vi "RecognitionSystem).vi"() -> ()   [LabVIEW 2011]
uses:
  <vilib>/DAQmx/read.llb/DAQmx Read (Digital Bool 1Line 1Point).vi
  <vilib>/DAQmx/write.llb/DAQmx Write (Digital Bool 1Line 1Point).vi
  <vilib>/DAQmx/create/channels.llb/DAQmx Create Channel (DI-Digital Input).vi
  <vilib>/DAQmx/create/channels.llb/DAQmx Create Channel (DO-Digital Output).vi
  <vilib>/DAQmx/miscellaneous.llb/DAQmx Fill In Error Info.vi
  <vilib>/Utility/file.llb/Read From Spreadsheet File (string).vi
  <vilib>/Utility/file.llb/Write To Spreadsheet File (string).vi
panel:
  in  "Tab Control":enum32{"System", "Sensors & Actuators"}(tab)
  in  "Data - File Path":path
  in  "Queue - File Path":path
  out "System Efficiency":dbl(knob) scale=0.0..100.0
  in  "Pause":bool
  out "Metal Count":dbl
  out "Plastic Count":dbl
  out "Dequeued Element":string
  out "# Elements in Queue":i32
  out "Hopper \nCount":i32(slide) scale=0.0..5.0
  in  "Stop GUI":bool
  out "Running":bool
  out "Stop":bool
  out "Belt & Chain":bool
  out "Assembled":dbl
  out "Efficiency":dbl
  out "Assembled":u8(slide) scale=0.0..10.0
  out "Plastics":u8(slide) scale=0.0..10.0
  out "Metals":u8(slide) scale=0.0..10.0
  out "Infrared Detector":bool
  out "Metal Detector":bool
  out "Sort Solenoid":bool=TRUE
  out "Assembly IR":bool
  out "Rotary Solenoid":bool=TRUE
  out "Reject IR":bool
  out "Sensing - Metal Detector":bool
  out "Capacitive Sensor":bool
  out "Fibre Optic":bool
  out "Reject Solenoid":bool
  out "Metal State":bool=TRUE
  out "Metal State 2":bool
  out "Capacitive State":bool=TRUE
  out "Sensing - Plastic State":bool
  out "Sort Solenoid Return":bool
  out "File Read":bool=TRUE
  out "Loop Iteration":i32
  out "Reject Solenoid Return":bool
  out "Reject IR - Neg Edge":bool
  out "Fibre Optic - Neg Edge":bool
  out "Pos Edge - Capacitive State":bool
  out "Pos Edge - Metal State 2":bool
  out "Fibre Optic Pos Edge":bool
  out "Capacitive - NEG Edge":bool
  out "Positive Edge - Rotary Solenoid":bool
  out "Reject IR - Pos Edge":bool
  out "IR Positive Edge":bool
  out "IR Negative Edge":bool
  # "Not Important Indicators"
  # "ICT Control System"
  # "Assembly Unit"
  # "Data Values"
  # "Rejecting Section"
  # "Sorting Section"
  # "Assembly Section"
  # "Sensing Section"
  # "Sort Solenoid Return"
  # "System States"
  # "File Read"
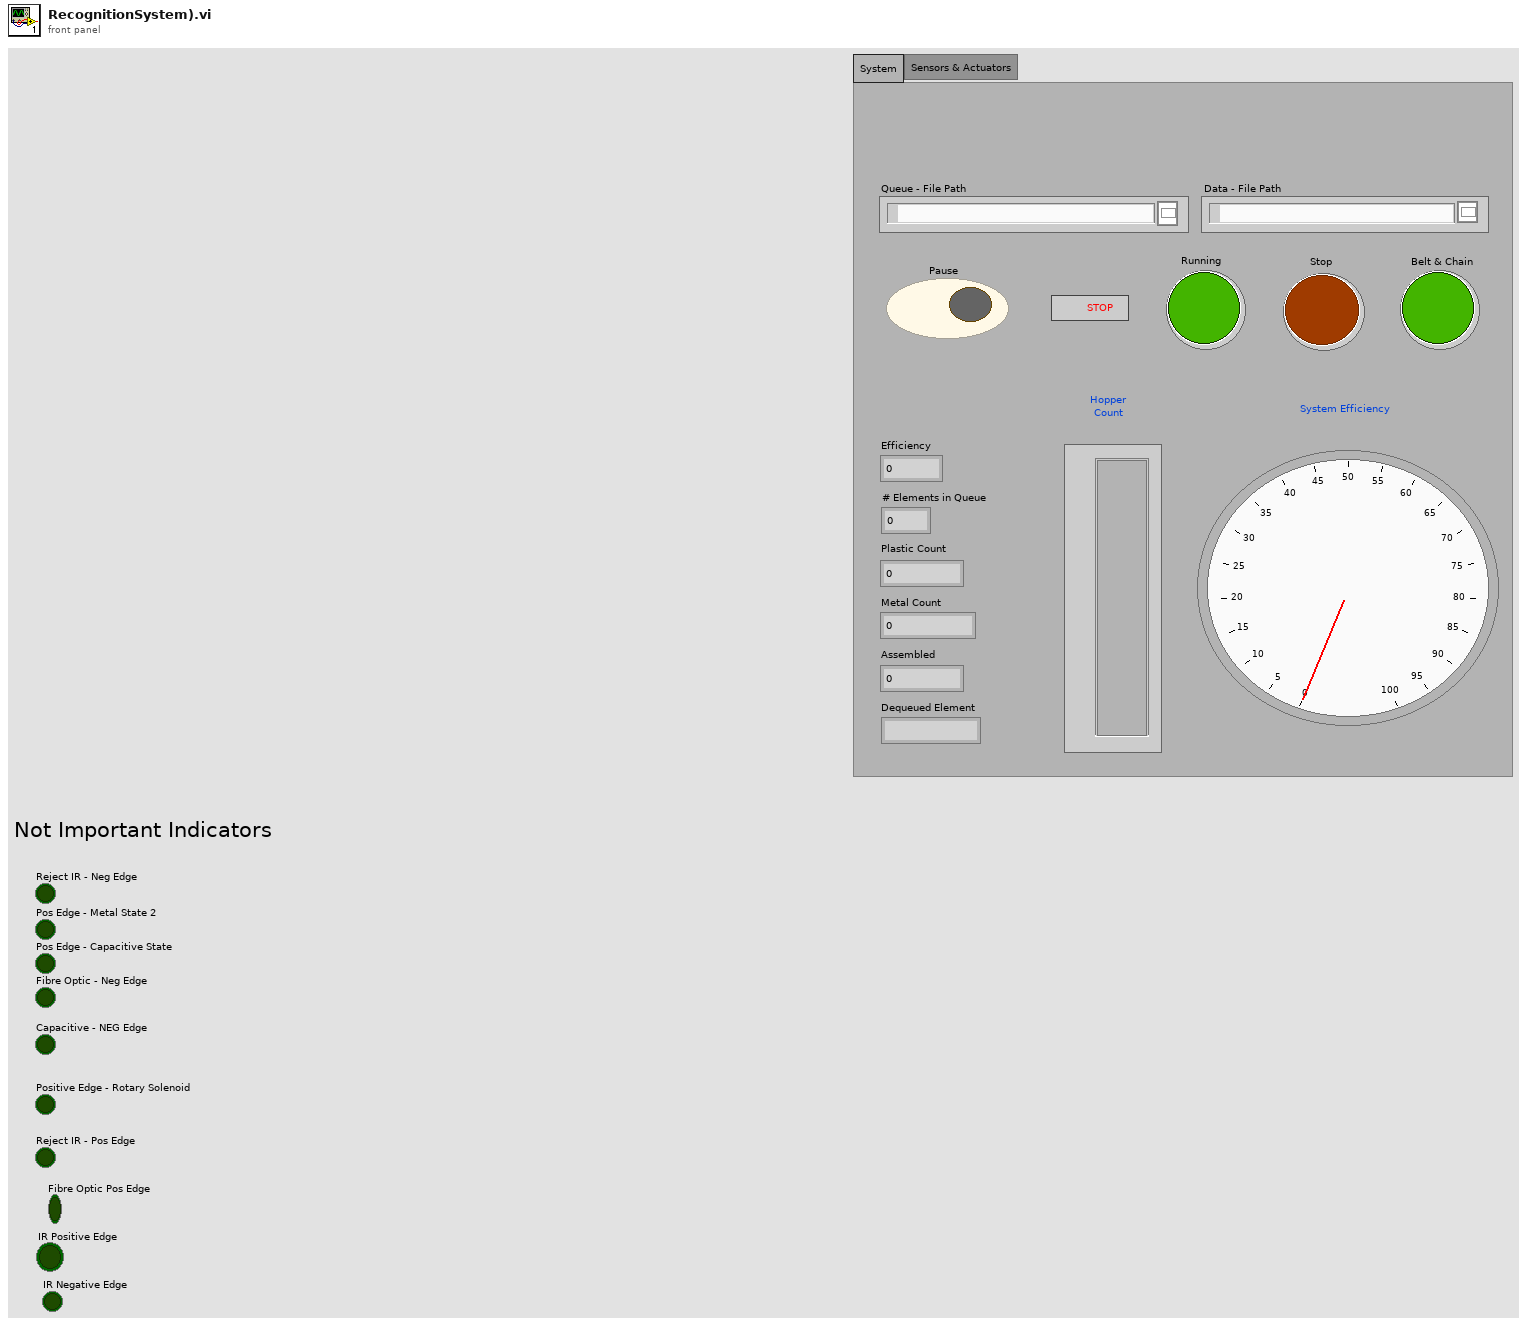
[diagram p1: front panel]
types:
  T1 = enum16{"open", "replace", "create", "open or create", "replace or create", "replace or create with confirmation"}
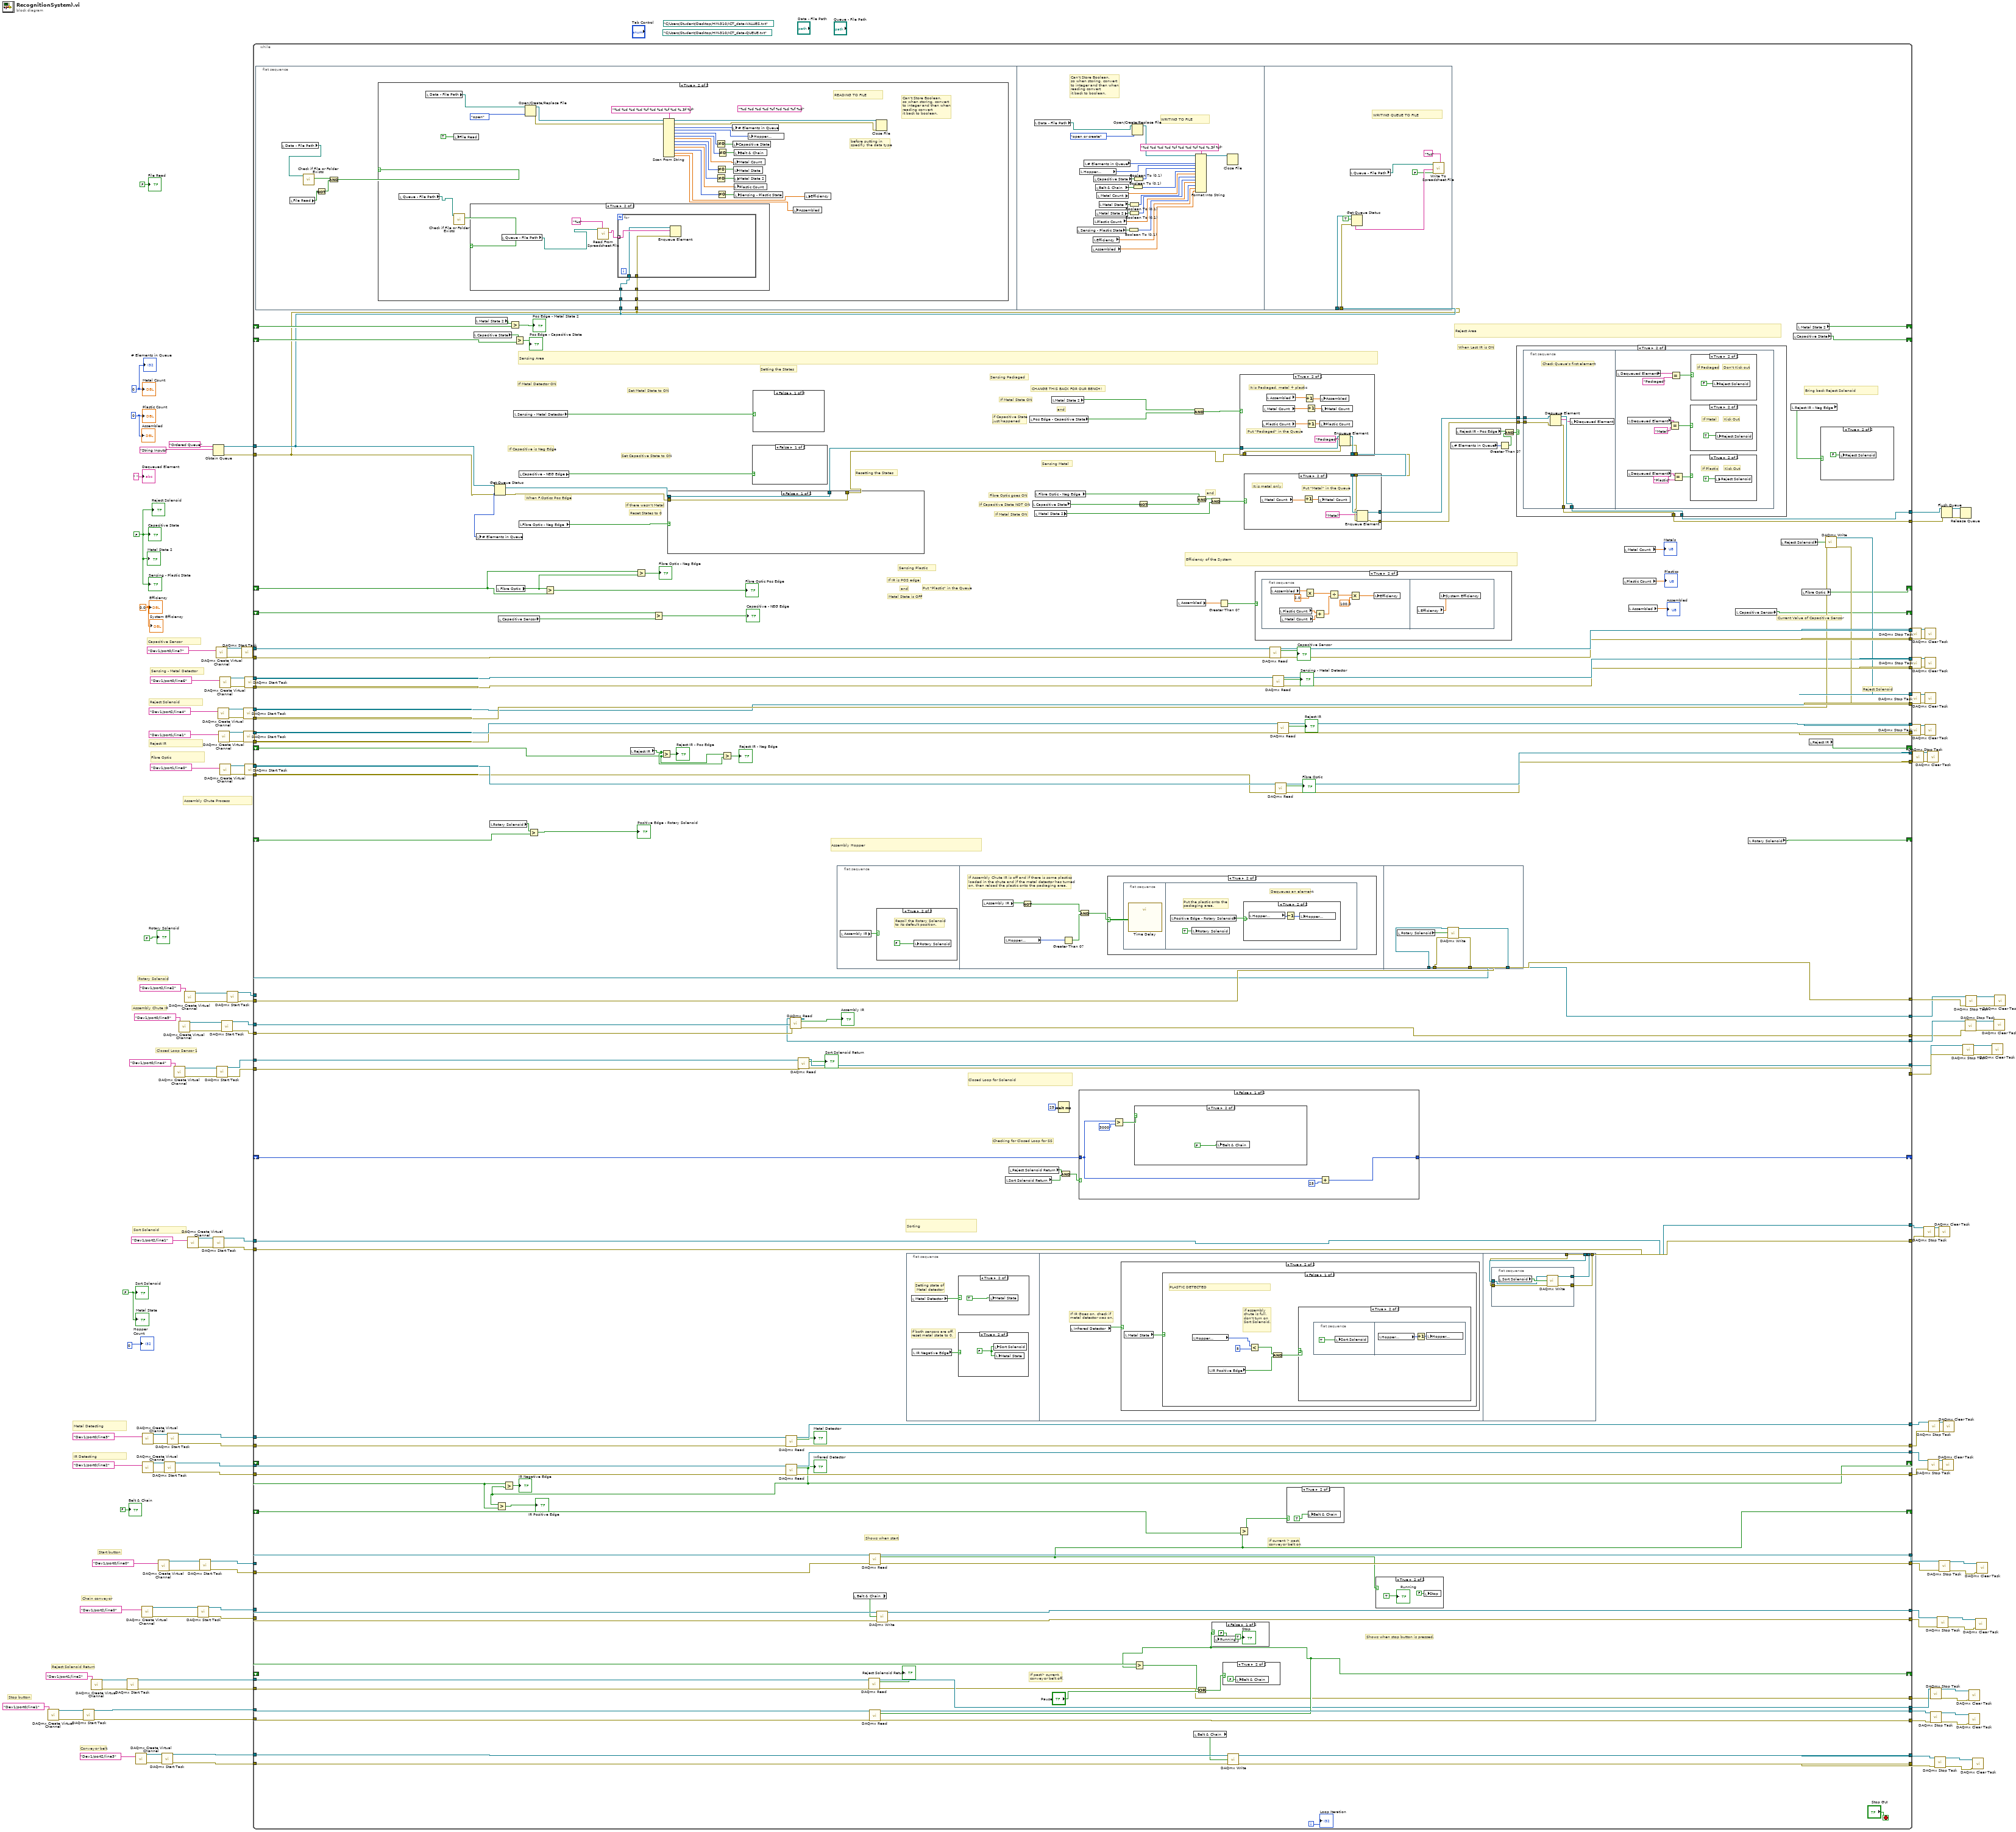
[diagram p0: block diagram]
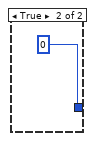
[diagram p3: hidden frame]
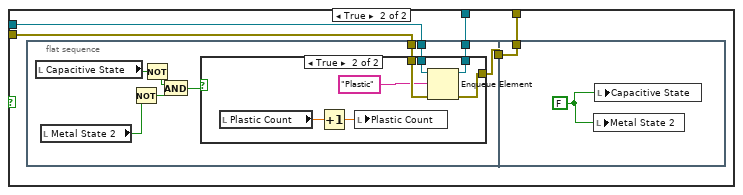
[diagram p16: hidden frame]
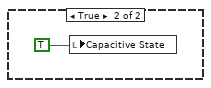
[diagram p18: hidden frame]
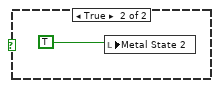
[diagram p19: hidden frame]
diagram:
  (unwired) path "C:/Users/Student/Desktop/HM-310/ICT_data-QUEUE.txt" ("file path (use dialog)")
  (unwired) path "C:/Users/Student/Desktop/HM-310/ICT_data-VALUES.txt" ("file path (use dialog)")
  w10 = 0.0 ("Efficiency")
  w12 = 0
  w15 = 0
  w26 = FALSE
  w25 = FALSE
  # "Reject Solenoid Return"
  # "Conveyor belt"
  # "Fibre Optic"
  # "Assembly Chute Process"
  # "Reject IR"
  # "Reject Solenoid"
  # "Sensing - Metal Detector"
  # "Capacitive Sensor"
  # "Rotary Solenoid"
  # "Assembly Chute IR"
  # "Closed Loop Sensor 1"
  # "Sort Solenoid"
  # "Chain conveyor"
  # "Stop button"
  # "Start button"
  # "IR Detecting"
  # "Metal Detecting"
  n1 = call-poly <vilib>:"DAQmx Create Virtual Channel.vi"("lines"=tag "Dev1/port0/line1") -> ("task out"=w111:refnum<k21>, "error out"=w119:errorcluster)  [unwired: 13 in]
  n2 = call <vilib>:"DAQmx Start Task.vi"("task/channels in"=w111, "error in"=w119) -> ("task out"=w117:refnum<k21>, "error out"=w116:errorcluster)  [unwired: 12 in]
  n3 = call-poly <vilib>:"DAQmx Create Virtual Channel.vi"("lines"=tag "Dev1/port1/line2") -> ("task out"=w7:refnum<k21>, "error out"=w9:errorcluster)  [unwired: 13 in]
  n4 = call <vilib>:"DAQmx Start Task.vi"("task/channels in"=w7, "error in"=w9) -> ("task out"=w2:refnum<k21>, "error out"=w1:errorcluster)  [unwired: 12 in]
  n5 = call-poly <vilib>:"DAQmx Create Virtual Channel.vi"("lines"=tag "Dev1/port2/line3") -> ("task out"=w36:refnum<k21>, "error out"=w35:errorcluster)  [unwired: 13 in]
  n6 = call-poly <vilib>:"DAQmx Create Virtual Channel.vi"("lines"=tag "Dev1/port2/line0") -> ("task out"=w128:refnum<k21>, "error out"=w127:errorcluster)  [unwired: 13 in]
  n7 = call-poly <vilib>:"DAQmx Create Virtual Channel.vi"("lines"=tag "Dev1/port0/line3") -> ("task out"=w161:refnum<k21>, "error out"=w160:errorcluster)  [unwired: 13 in]
  n8 = call-poly <vilib>:"DAQmx Create Virtual Channel.vi"("lines"=tag "Dev1/port0/line2") -> ("task out"=w147:refnum<k21>, "error out"=w146:errorcluster)  [unwired: 13 in]
  n9 = call-poly <vilib>:"DAQmx Create Virtual Channel.vi"("lines"=tag "Dev1/port0/line0") -> ("task out"=w136:refnum<k21>, "error out"=w135:errorcluster)  [unwired: 13 in]
  n10 = call <vilib>:"DAQmx Start Task.vi"("task/channels in"=w36, "error in"=w35) -> ("task out"=w33:refnum<k21>, "error out"=w32:errorcluster)  [unwired: 12 in]
  n11 = call <vilib>:"DAQmx Start Task.vi"("task/channels in"=w147, "error in"=w146) -> ("task out"=w141:refnum<k21>, "error out"=w140:errorcluster)  [unwired: 12 in]
  n12 = call <vilib>:"DAQmx Start Task.vi"("task/channels in"=w161, "error in"=w160) -> ("task out"=w150:refnum<k21>, "error out"=w149:errorcluster)  [unwired: 12 in]
  n13 = call-poly <vilib>:"DAQmx Create Virtual Channel.vi"("lines"=tag "Dev1/port0/line4") -> ("task out"=w108:refnum<k21>, "error out"=w107:errorcluster)  [unwired: 13 in]
  n14 = call-poly <vilib>:"DAQmx Create Virtual Channel.vi"("lines"=tag "Dev1/port0/line5") -> ("task out"=w99:refnum<k21>, "error out"=w98:errorcluster)  [unwired: 13 in]
  n15 = call-poly <vilib>:"DAQmx Create Virtual Channel.vi"("lines"=tag "Dev1/port2/line2") -> ("task out"=w88:refnum<k21>, "error out"=w87:errorcluster)  [unwired: 13 in]
  n16 = call-poly <vilib>:"DAQmx Create Virtual Channel.vi"("lines"=tag "Dev1/port2/line1") -> ("task out"=w157:refnum<k21>, "error out"=w156:errorcluster)  [unwired: 13 in]
  n17 = call <vilib>:"DAQmx Start Task.vi"("task/channels in"=w128, "error in"=w127) -> ("task out"=w125:refnum<k21>, "error out"=w124:errorcluster)  [unwired: 12 in]
  n18 = call <vilib>:"DAQmx Start Task.vi"("task/channels in"=w136, "error in"=w135) -> ("task out"=w134:refnum<k21>, "error out"=w133:errorcluster)  [unwired: 12 in]
  n19 = Obtain Queue(name (unnamed)="Ordered Queue", element data type="String Inputs") -> (queue out=w22:refnum<queue>, error out=w21:errorcluster)  [unwired: 3 in, 1 out]
  n20 = call <vilib>:"DAQmx Start Task.vi"("task/channels in"=w157, "error in"=w156) -> ("task out"=w139:refnum<k21>, "error out"=w138:errorcluster)  [unwired: 12 in]
  n21 = call-poly <vilib>:"DAQmx Create Virtual Channel.vi"("lines"=tag "Dev1/port0/line7") -> ("task out"=w80:refnum<k21>, "error out"=w79:errorcluster)  [unwired: 13 in]
  n22 = call <vilib>:"DAQmx Start Task.vi"("task/channels in"=w108, "error in"=w107) -> ("task out"=w105:refnum<k21>, "error out"=w104:errorcluster)  [unwired: 12 in]
  n23 = call-poly <vilib>:"DAQmx Create Virtual Channel.vi"("lines"=tag "Dev1/port2/line4") -> ("task out"=w74:refnum<k21>, "error out"=w73:errorcluster)  [unwired: 13 in]
  n24 = call-poly <vilib>:"DAQmx Create Virtual Channel.vi"("lines"=tag "Dev1/port1/line1") -> ("task out"=w71:refnum<k21>, "error out"=w70:errorcluster)  [unwired: 13 in]
  n25 = call-poly <vilib>:"DAQmx Create Virtual Channel.vi"("lines"=tag "Dev1/port0/line6") -> ("task out"=w77:refnum<k21>, "error out"=w76:errorcluster)  [unwired: 13 in]
  n26 = call-poly <vilib>:"DAQmx Create Virtual Channel.vi"("lines"=tag "Dev1/port1/line0") -> ("task out"=w60:refnum<k21>, "error out"=w59:errorcluster)  [unwired: 13 in]
  n27 = call <vilib>:"DAQmx Start Task.vi"("task/channels in"=w99, "error in"=w98) -> ("task out"=w96:refnum<k21>, "error out"=w95:errorcluster)  [unwired: 12 in]
  n28 = call <vilib>:"DAQmx Start Task.vi"("task/channels in"=w88, "error in"=w87) -> ("task out"=w85:refnum<k21>, "error out"=w84:errorcluster)  [unwired: 12 in]
  n29 = call <vilib>:"DAQmx Start Task.vi"("task/channels in"=w80, "error in"=w79) -> ("task out"=w69:refnum<k21>, "error out"=w68:errorcluster)  [unwired: 12 in]
  n30 = call <vilib>:"DAQmx Start Task.vi"("task/channels in"=w74, "error in"=w73) -> ("task out"=w65:refnum<k21>, "error out"=w64:errorcluster)  [unwired: 12 in]
  n31 = call <vilib>:"DAQmx Start Task.vi"("task/channels in"=w71, "error in"=w70) -> ("task out"=w63:refnum<k21>, "error out"=w62:errorcluster)  [unwired: 12 in]
  n32 = call <vilib>:"DAQmx Start Task.vi"("task/channels in"=w77, "error in"=w76) -> ("task out"=w67:refnum<k21>, "error out"=w66:errorcluster)  [unwired: 12 in]
  n33 = call <vilib>:"DAQmx Start Task.vi"("task/channels in"=w60, "error in"=w59) -> ("task out"=w58:refnum<k21>, "error out"=w57:errorcluster)  [unwired: 12 in]
  n34 = while {
    tunnel: [w318] -> w152
    tunnel: [w317] -> w151
    tunnel: w150 -> [w316]
    tunnel: w149 -> [w315]
    tunnel: [w314] -> w143
    tunnel: [w313] -> w142
    tunnel: w141 -> [w312]
    tunnel: w140 -> [w311]
    tunnel: w139 -> [w281]
    tunnel: w138 -> [w280]
    tunnel: w134 -> [w308]
    tunnel: w133 -> [w307]
    tunnel: [w306] -> w130
    tunnel: [w305] -> w129
    tunnel: w125 -> [w304]
    tunnel: w124 -> [w303]
    tunnel: [w302] -> w121
    tunnel: [w301] -> w120
    tunnel: w117 -> [w300]
    tunnel: w116 -> [w299]
    tunnel: [w298] -> w113
    tunnel: [w297] -> w112
    shift-right: [w178] -> _
    shift-left: _ -> [w296]
    shift-right: [w179] -> _
    shift-left: _ -> [w294]
    tunnel: [w283] -> w101
    shift-right: [w285] -> _
    shift-left: _ -> [w286]
    tunnel: w105 -> [w291]
    tunnel: w104 -> [w290]
    tunnel: [w289] -> w103
    tunnel: [w288] -> w102
    tunnel: [w282] -> w100
    tunnel: w96 -> [w279]
    tunnel: w95 -> [w278]
    tunnel: [w277] -> w92
    tunnel: [w276] -> w91
    tunnel: w85 -> [w271]
    tunnel: w84 -> [w273]
    tunnel: [w274] -> w83
    tunnel: [w272] -> w82
    tunnel: w69 -> [w263]
    tunnel: w68 -> [w264]
    tunnel: w67 -> [w265]
    tunnel: w66 -> [w266]
    tunnel: w65 -> [w267]
    tunnel: w64 -> [w268]
    tunnel: w63 -> [w270]
    tunnel: w62 -> [w269]
    tunnel: w58 -> [w262]
    tunnel: w57 -> [w261]
    tunnel: [w260] -> w38
    tunnel: [w259] -> w37
    tunnel: [w258] -> w40
    tunnel: [w257] -> w39
    tunnel: [w256] -> w42
    tunnel: [w255] -> w41
    tunnel: [w254] -> w44
    tunnel: [w253] -> w43
    tunnel: [w252] -> w46
    tunnel: [w251] -> w45
    tunnel: w33 -> [w247]
    tunnel: w32 -> [w246]
    tunnel: [w244] -> w29
    tunnel: [w243] -> w28
    shift-right: [w200] -> _
    shift-left: _ -> [w194]
    shift-right: [w237] -> _
    shift-left: _ -> [w236]
    shift-right: [w233] -> _
    shift-left: _ -> [w229]
    shift-right: [w231] -> _
    shift-left: _ -> [w209]
    shift-right: [w221] -> _
    shift-left: _ -> [w220]
    shift-right: [w217] -> _
    shift-left: _ -> [w216]
    tunnel: w22 -> [w183]
    tunnel: w21 -> [w182]
    tunnel: [w196] -> w20
    tunnel: [w197] -> w17
    shift-right: [w175] -> _
    shift-left: _ -> [w176]
    tunnel: [w173] -> w4
    tunnel: [w172] -> w3
    tunnel: w2 -> [w171]
    tunnel: w1 -> [w170]
    i -> [w174]
    stop <- "Stop GUI" stop-if-true
    # "Bring back Reject Solenoid"
    # "Efficiency of the System"
    # "Closed Loop for Solenoid"
    # "Sorting"
    # "Assembly Hopper"
    # "Checking for Closed Loop for SS"
    # "When Last IR is ON"
    # "CHANGE THIS BACK FOR OUR BENCH!"
    # "Fibre Optic goes ON"
    # "and"
    # "Sensing Packaged"
    # "if Capacitive State \njust happened"
    # "If Metal State ON"
    # "and"
    # "Sensing Plastic"
    # "Sensing Metal"
    # "Put \"Plastic\" in the Queue"
    # "Metal State is OFF"
    # "and"
    # "If IR is POS edge"
    # "If Capacitive State NOT ON"
    # "If Metal State ON"
    # "If there wasn't Metal"
    # "Set Capacitive State to ON"
    # "If Capacitive is Neg Edge"
    # "Resetting the States"
    # "Setting the States"
    # "Reset States to 0"
    # "When F.Optics Pos Edge"
    # "Set Metal State to ON"
    # "If Metal Detector ON"
    # "Current Value of Capacitive Sensor"
    # "Reject Solenoid"
    # "Reject Area"
    # "Sensing Area"
    # "Shows when stop button is pressed."
    # "If past> current,\nconveyor belt off."
    # "If current > past,\nconveyor belt on"
    # "Shows when start"
    n35 = flat-sequence {
      tunnel: w183 -> [w342]
      tunnel: w182 -> [w341]
      tunnel: w182 -> [w407]
      tunnel: w183 -> [w408]
      frame #0 {
        n36 = local read "Data - File Path"() -> (w340:path)
        n37 = local read "File Read"() -> (w344:bool)
        n38 = call <vilib>:"Check if File or Folder Exists.vi"("path"=w340) -> ("file or folder exists?"=w345:bool)  [unwired: 8 in, 2 out]
        n39 = Not(x=w344) -> (.not. x?=w343:bool)
        n40 = And(x=w345, y=w343) -> (x .and. y?=w346:bool)
        n41 = case shown="True" w346 {
          tunnel: w342 -> [_ w352]
          tunnel: w341 -> [_ w351]
          frame False {
          }
          frame True {
            (unwired) "%d %d %d %d %f %d %d %f %d" ("format string")
            # "before putting in \nspecifiy the data type"
            # "Can't Store Boolean,\nso when storing, convert \nto integer and then when \nreading convert\nit back to boolean."
            # "READING TO FILE"
            n42 = local read "Queue - File Path"() -> (w347:path)
            n43 = local read "Data - File Path"() -> (w348:path)
            n44 = local write "File Read"(TRUE) -> ()
            n45 = call <vilib>:"Check if File or Folder Exists.vi"("path"=w347) -> ("file or folder exists?"=w353:bool)  [unwired: 8 in, 2 out]
            n46 = case shown="True" w353 {
              tunnel: w352 -> [_ w376]
              tunnel: w351 -> [_ w377]
              frame False {
              }
              frame True {
                n47 = local read "Queue - File Path"() -> (w375:path)
                n48 = call-poly <vilib>:"Read From Spreadsheet File.vi"("format (%s)"="%s", "file path (dialog if empty)"=w375) -> ("first row"=w378:string[])  [unwired: 5 in, 4 out]
                n49 = for {
                  tunnel: w378 -> [w382] mode=indexing
                  tunnel: w377 -> [w381]
                  tunnel: w376 -> [w380]
                  n50 = Enqueue Element(queue=w380, element=w382, error in (no error)=w381) -> ()  [unwired: 1 in, 3 out]
                }
              }
            }
            n51 = Open/Create/Replace File(file path (use dialog)=w348, operation (0:open)=T1."open") -> (refnum out=w373:refnum<file>, error out=w372:errorcluster)  [unwired: 4 in, 1 out]
            n52 = Scan From String("%d %d %d %d %f %d %d %f %d %.3f %f" ("format string"), w373, w372) -> (w356:refnum<file>, w355:errorcluster, output 1=w371:i32, output 2=w370:i32, output 3=w368:i32, output 4=w357:i32, output 5=w362:dbl, output 6=w361:i32, output 7=w360:i32, output 8=w359:dbl, output 9=w358:i32, output 10=w350:dbl, output 11=w349:dbl)  [unwired: 11 in]
            n53 = Not Equal To 0?(x=w368) -> (x != 0?=w369:bool)
            n54 = Not Equal To 0?(x=w360) -> (x != 0?=w364:bool)
            n55 = Not Equal To 0?(x=w361) -> (x != 0?=w365:bool)
            n56 = Not Equal To 0?(x=w358) -> (x != 0?=w363:bool)
            n57 = Not Equal To 0?(x=w357) -> (x != 0?=w366:bool)
            n58 = local write "# Elements in Queue"(w371) -> ()
            n59 = local write "Capacitive State"(w369) -> ()
            n60 = local write "Metal Count"(w362) -> ()
            n61 = local write "Metal State"(w365) -> ()
            n62 = local write "Metal State 2"(w364) -> ()
            n63 = local write "Plastic Count"(w359) -> ()
            n64 = local write "Belt & Chain"(w366) -> ()
            n65 = local write "Sensing - Plastic State"(w363) -> ()
            n66 = local write "Hopper \nCount"(w370) -> ()
            n67 = local write "Assembled"(w349) -> ()
            n68 = local write "Efficiency"(w350) -> ()
            n69 = Close File(refnum=w356, error in=w355) -> ()  [unwired: 2 out]
          }
        }
      }
      frame #1 {
        # "Can't Store Boolean,\nso when storing, convert \nto integer and then when \nreading convert\nit back to boolean."
        # "WRITING TO FILE"
        n70 = local read "Data - File Path"() -> (w383:path)
        n71 = local read "Sensing - Plastic State"() -> (w396:bool)
        n72 = local read "Hopper \nCount"() -> (w399:i32)
        n73 = local read "# Elements in Queue"() -> (w386:i32)
        n74 = local read "Assembled"() -> (w384:dbl)
        n75 = local read "Efficiency"() -> (w385:dbl)
        n76 = local read "Capacitive State"() -> (w388:bool)
        n77 = local read "Plastic Count"() -> (w397:dbl)
        n78 = local read "Belt & Chain"() -> (w389:bool)
        n79 = local read "Metal State 2"() -> (w394:bool)
        n80 = local read "Metal Count"() -> (w391:dbl)
        n81 = local read "Metal State"() -> (w392:bool)
        n82 = Boolean To (0,1)(Boolean=w396) -> (0, 1=w398:i16)
        n83 = Boolean To (0,1)(Boolean=w392) -> (0, 1=w393:i16)
        n84 = Boolean To (0,1)(Boolean=w394) -> (0, 1=w395:i16)
        n85 = Open/Create/Replace File(file path (use dialog)=w383, operation (0:open)=T1."open or create") -> (refnum out=w402:refnum<file>)  [unwired: 4 in, 2 out]
        n86 = Boolean To (0,1)(Boolean=w389) -> (0, 1=w390:i16)
        n87 = Boolean To (0,1)(Boolean=w388) -> (0, 1=w400:i16)
        n88 = Format Into String(format string="%d %d %d %d %f %d %d %f %d %.3f %f", initial string=w402, w386, w399, w400, w390, w391, w393, w395, w397, w398, w385, w384) -> (resulting string=w403:refnum<file>)  [unwired: 1 in, 1 out]
        n89 = Close File(refnum=w403) -> ()  [unwired: 1 in, 2 out]
      }
      frame #2 {
        # "WRITING QUEUE TO FILE"
        n90 = local read "Queue - File Path"() -> (w404:path)
        n91 = Get Queue Status(queue=w408, return elements? (F)=TRUE, error in (no error)=w407) -> (elements=w410:string[])  [unwired: 7 out]
        n92 = call-poly <vilib>:"Write To Spreadsheet File.vi"("format (%s)"="%s", "append to file? (new file:F)"=FALSE, "1D data"=w410, "file path (dialog if empty)"=w404) -> ()  [unwired: 4 in, 1 out]
      }
    }
    n93 = local read "Capacitive State"() -> (w215:bool)
    n94 = local read "Metal State 2"() -> (w219:bool)
    n95 = local read "Rotary Solenoid"() -> (w235:bool)
    n96 = Get Queue Status(queue=w183, error in (no error)=w182) -> (queue out=w190:refnum<queue>, error out=w189:errorcluster, # elements in queue=w188:i32)  [unwired: 1 in, 5 out]
    n97 = local write "# Elements in Queue"(w188) -> ()
    n98 = local read "Fibre Optic"() -> (w210:bool)
    n99 = local read "Capacitive Sensor"() -> (w230:bool)
    n100 = Greater?(x=w219, y=w220) -> (0:→"Pos Edge - Metal State 2":bool)
    n101 = local read "Sensing - Metal Detector"() -> (w227:bool)
    n102 = Greater?(x=w215, y=w216) -> (0:→"Pos Edge - Capacitive State":bool)
    n103 = local read "Capacitive - NEG Edge"() -> (w226:bool)
    n104 = local read "Fibre Optic - Neg Edge"() -> (w225:bool)
    n105 = Greater?(x=w235, y=w236) -> (0:→"Positive Edge - Rotary Solenoid":bool)
    n106 = Greater?(x=w210, y=w209) -> (0:→"Fibre Optic Pos Edge":bool)
    n107 = local read "Reject IR"() -> (w195:bool)
    n108 = Greater?(x=w209, y=w210) -> (0:→"Fibre Optic - Neg Edge":bool)
    n109 = Greater?(x=w229, y=w230) -> (0:→"Capacitive - NEG Edge":bool)
    n110 = Greater?(x=w195, y=w194) -> (0:→"Reject IR - Pos Edge":bool)
    n111 = case shown="False" w225 {
      tunnel: w190 -> [w458 w463]
      tunnel: w189 -> [w457 w462]
      tunnel: [w458 w461] -> w204
      tunnel: [w457 w459] -> w201
      frame False {
      }
      frame True {
        n112 = flat-sequence {
          tunnel: w463 -> [w467]
          tunnel: w462 -> [w466]
          tunnel: [w465] -> w461
          tunnel: [w464] -> w460
          tunnel: w460 -> [w482]
          tunnel: [w482] -> w459
          frame #0 {
            n113 = local read "Capacitive State"() -> (w469:bool)
            n114 = local read "Metal State 2"() -> (w471:bool)
            n115 = Not(x=w471) -> (.not. x?=w470:bool)
            n116 = Not(x=w469) -> (.not. x?=w468:bool)
            n117 = And(x=w468, y=w470) -> (x .and. y?=w472:bool)
            n118 = case shown="True" w472 {
              tunnel: w467 -> [w474 w479]
              tunnel: w466 -> [w473 w478]
              tunnel: [w474 w476] -> w465
              tunnel: [w473 w475] -> w464
              frame False {
              }
              frame True {
                n119 = local read "Plastic Count"() -> (w480:dbl)
                n120 = Increment(x=w480) -> (x+1=w481:dbl)
                n121 = local write "Plastic Count"(w481) -> ()
                n122 = Enqueue Element(queue=w479, element="Plastic", error in (no error)=w478) -> (queue out=w476:refnum<queue>, error out=w475:errorcluster)  [unwired: 1 in, 1 out]
              }
            }
          }
          frame #1 {
            w483 = FALSE
            n123 = local write "Metal State 2"(w483) -> ()
            n124 = local write "Capacitive State"(w483) -> ()
          }
        }
      }
    }
    n125 = Greater?(x=w194, y=w195) -> (0:→"Reject IR - Neg Edge":bool)
    n126 = case shown="False" w226 {
      frame False {
      }
      frame True {
        n127 = local write "Capacitive State"(TRUE) -> ()
      }
    }
    n128 = case shown="False" w227 {
      frame False {
      }
      frame True {
        n129 = local write "Metal State 2"(TRUE) -> ()
      }
    }
    n130 = call-poly <vilib>:"DAQmx Read.vi"("task/channels in"=w316, "error in"=w315) -> ("task out"=w317:refnum<k21>, "data"=→"Metal Detector":bool, "error out"=w318:errorcluster)  [unwired: 11 in]
    n131 = call-poly <vilib>:"DAQmx Read.vi"("task/channels in"=w312, "error in"=w311) -> ("task out"=w313:refnum<k21>, "data"=w285:bool, "error out"=w314:errorcluster)  [unwired: 11 in]
    "Infrared Detector" <- w285
    n132 = Greater?(x=w285, y=w286) -> (0:→"IR Positive Edge":bool)
    n133 = Greater?(x=w286, y=w285) -> (0:→"IR Negative Edge":bool)
    n134 = call-poly <vilib>:"DAQmx Read.vi"("task/channels in"=w279, "error in"=w278) -> ("task out"=w277:refnum<k21>, "data"=→"Assembly IR":bool, "error out"=w276:errorcluster)  [unwired: 11 in]
    n135 = call-poly <vilib>:"DAQmx Read.vi"("task/channels in"=w291, "error in"=w290) -> ("task out"=w288:refnum<k21>, "data"=→"Sort Solenoid Return":bool, "error out"=w289:errorcluster)  [unwired: 11 in]
    n136 = flat-sequence {
      tunnel: w271 -> [w501]
      tunnel: [w500] -> w274
      tunnel: [w499] -> w272
      tunnel: w273 -> [w498]
      frame #0 {
        n137 = local read "Assembly IR"() -> (w486:bool)
        n138 = case shown="True" w486 {
          frame False {
          }
          frame True {
            # "Recoil the Rotary Solenoid\nto its default position."
            n139 = local write "Rotary Solenoid"(FALSE) -> ()
          }
        }
      }
      frame #1 {
        # "If Assembly Chute IR is off and if there is some plastics\nloaded in the chute and if the metal detector has turned\non, then reload the plastic onto the packaging area."
        n140 = local read "Assembly IR"() -> (w492:bool)
        n141 = local read "Hopper \nCount"() -> (w490:i32)
        n142 = Not(x=w492) -> (.not. x?=w491:bool)
        n143 = Greater Than 0?(x=w490) -> (x > 0?=w489:bool)
        n144 = And(x=w491, y=w489) -> (x .and. y?=w488:bool)
        n145 = case shown="True" w488 {
          frame False {
          }
          frame True {
            n146 = flat-sequence {
              frame #0 {
                n147 = call "Time Delay"() -> ()  [unwired: 11 in, 1 out]
              }
              frame #1 {
                # "Dequeues an element"
                # "Put the plastic onto the \npackaging area."
                n148 = local read "Positive Edge - Rotary Solenoid"() -> (w494:bool)
                n149 = local write "Rotary Solenoid"(TRUE) -> ()
                n150 = case shown="True" w494 {
                  frame False {
                  }
                  frame True {
                    n151 = local read "Hopper \nCount"() -> (w496:i32)
                    n152 = Decrement(x=w496) -> (x-1=w495:i32)
                    n153 = local write "Hopper \nCount"(w495) -> ()
                  }
                }
              }
            }
          }
        }
      }
      frame #2 {
        n154 = local read "Rotary Solenoid"() -> (w497:bool)
        n155 = call-poly <vilib>:"DAQmx Write.vi"("task/channels in"=w501, "data"=w497, "error in"=w498) -> ("task out"=w499:refnum<k21>, "error out"=w500:errorcluster)  [unwired: 10 in, 1 out]
      }
    }
    n156 = local read "Belt & Chain"() -> (w293:bool)
    n157 = call-poly <vilib>:"DAQmx Read.vi"("task/channels in"=w171, "error in"=w170) -> ("task out"=w173:refnum<k21>, "data"=→"Reject Solenoid Return":bool, "error out"=w172:errorcluster)  [unwired: 11 in]
    n158 = call-poly <vilib>:"DAQmx Read.vi"("task/channels in"=w308, "error in"=w307) -> ("task out"=w306:refnum<k21>, "data"=w179:bool, "error out"=w305:errorcluster)  [unwired: 11 in]
    n159 = call-poly <vilib>:"DAQmx Read.vi"("task/channels in"=w300, "error in"=w299) -> ("task out"=w298:refnum<k21>, "data"=w178:bool, "error out"=w297:errorcluster)  [unwired: 11 in]
    n160 = call-poly <vilib>:"DAQmx Write.vi"("task/channels in"=w304, "data"=w293, "error in"=w303) -> ("task out"=w302:refnum<k21>, "error out"=w301:errorcluster)  [unwired: 10 in, 1 out]
    n161 = flat-sequence {
      tunnel: [w519] -> w283
      tunnel: [w518] -> w282
      tunnel: w281 -> [w517]
      tunnel: w280 -> [w516]
      frame #0 {
        # "If both sensors are off, \nreset metal state to 0."
        # "Setting state of\n Metal detector"
        n162 = local read "Metal Detector"() -> (w503:bool)
        n163 = local read "IR Negative Edge"() -> (w502:bool)
        n164 = case shown="True" w502 {
          frame False {
          }
          frame True {
            w504 = FALSE
            n165 = local write "Sort Solenoid"(w504) -> ()
            n166 = local write "Metal State"(w504) -> ()
          }
        }
        n167 = case shown="True" w503 {
          frame False {
          }
          frame True {
            n168 = local write "Metal State"(TRUE) -> ()
          }
        }
      }
      frame #1 {
        # "If IR Goes on, check if \nmetal detector was on."
        n169 = local read "Infrared Detector"() -> (w506:bool)
        n170 = case shown="True" w506 {
          frame False {
          }
          frame True {
            n171 = local read "Metal State"() -> (w507:bool)
            n172 = case shown="False" w507 {
              frame False {
                # "if assembly\nchute is full, \ndon't turn on \nSort Solenoid."
                # "PLASTIC DETECTED"
                n173 = local read "Hopper \nCount"() -> (w511:i32)
                n174 = local read "IR Positive Edge"() -> (w508:bool)
                n175 = Less?(x=w511, y=5) -> (x < y?=w509:bool)
                n176 = And(x=w509, y=w508) -> (x .and. y?=w512:bool)
                n177 = case shown="True" w512 {
                  frame False {
                  }
                  frame True {
                    n178 = flat-sequence {
                      frame #0 {
                        n179 = local write "Sort Solenoid"(TRUE) -> ()
                      }
                      frame #1 {
                        n180 = local read "Hopper \nCount"() -> (w515:i32)
                        n181 = Increment(x=w515) -> (x+1=w514:i32)
                        n182 = local write "Hopper \nCount"(w514) -> ()
                      }
                    }
                  }
                }
              }
              frame True {
                # "Count metal, let it go.. let it goooo, let it gooooo"
              }
            }
          }
        }
      }
      frame #2 {
        n183 = flat-sequence {
          tunnel: w516 -> [w520]
          tunnel: w517 -> [w521]
          tunnel: [w522] -> w518
          tunnel: [w523] -> w519
          frame #0 {
            n184 = local read "Sort Solenoid"() -> (w524:bool)
            n185 = call-poly <vilib>:"DAQmx Write.vi"("task/channels in"=w521, "data"=w524, "error in"=w520) -> ("task out"=w522:refnum<k21>, "error out"=w523:errorcluster)  [unwired: 10 in, 1 out]
          }
        }
      }
    }
    n186 = local read "Sort Solenoid Return"() -> (w166:bool)
    n187 = local read "Reject Solenoid Return"() -> (w167:bool)
    n188 = local read "Pos Edge - Capacitive State"() -> (w212:bool)
    n189 = local read "Capacitive State"() -> (w222:bool)
    n190 = local read "Metal State 2"() -> (w205:bool)
    n191 = local read "Fibre Optic - Neg Edge"() -> (w224:bool)
    n192 = local read "Metal State 2"() -> (w213:bool)
    n193 = Wait (ms)(milliseconds to wait=u32 25) -> ()  [unwired: 1 out]
    n194 = And(x=w167, y=w166) -> (x .and. y?=w168:bool)
    n195 = case shown="False" w168 {
      tunnel: w176 -> [w321 _]
      tunnel: [w322 u32 0 ("milliseconds to wait")] -> w175
      frame False {
        n196 = Greater?(x=w321, y=u32 3000) -> (0:w319:bool)
        n197 = case shown="True" w319 {
          frame False {
          }
          frame True {
            n198 = local write "Belt & Chain"(FALSE) -> ()
          }
        }
        n199 = Add(x=w321, y=u32 25 ("milliseconds to wait")) -> (x+y=w322:u32)
      }
      frame True {
      }
    }
    n200 = Greater?(x=w296, y=w178) -> (0:w240:bool)
    n201 = Not(x=w222) -> (.not. x?=w223:bool)
    n202 = local read "Assembled"() -> (w180:dbl)
    n203 = And(x=w213, y=w212) -> (x .and. y?=w211:bool)
    n204 = local read "Belt & Chain"() -> (w245:bool)
    n205 = And(x=w224, y=w223) -> (x .and. y?=w207:bool)
    n206 = Or(x=w240, y="Pause") -> (x .or. y?=w238:bool)
    n207 = And(x=w207, y=w205) -> (x .and. y?=w206:bool)
    n208 = case shown="False" w178 {
      frame False {
        n209 = local write "Running"(FALSE) -> ()
        "Stop" <- TRUE
      }
      frame True {
      }
    }
    n210 = Greater Than 0?(x=w180) -> (x > 0?=w181:bool)
    n211 = case shown="True" w238 {
      frame False {
      }
      frame True {
        n212 = local write "Belt & Chain"(FALSE ("Start")) -> ()
      }
    }
    n213 = call-poly <vilib>:"DAQmx Write.vi"("task/channels in"=w247, "data"=w245, "error in"=w246) -> ("task out"=w244:refnum<k21>, "error out"=w243:errorcluster)  [unwired: 10 in, 1 out]
    n214 = Greater?(x=w179, y=w294) -> (0:w295:bool)
    n215 = case shown="True" w211 {
      tunnel: w204 -> [w436 w442]
      tunnel: [w436 w441] -> w203
      tunnel: [w435 w440] -> w202
      tunnel: w201 -> [w435 w439]
      frame False {
      }
      frame True {
        # "Put \"Packaged\" in the Queue"
        # "It is Packaged, metal + plastic"
        n216 = local read "Plastic Count"() -> (w447:dbl)
        n217 = local read "Metal Count"() -> (w444:dbl)
        n218 = local read "Assembled"() -> (w438:dbl)
        n219 = Increment(x=w438) -> (x+1=w437:dbl)
        n220 = Increment(x=w444) -> (x+1=w445:dbl)
        n221 = Increment(x=w447) -> (x+1=w446:dbl)
        n222 = local write "Plastic Count"(w446) -> ()
        n223 = local write "Assembled"(w437) -> ()
        n224 = local write "Metal Count"(w445) -> ()
        n225 = Enqueue Element(queue=w442, element="Packaged", error in (no error)=w439) -> (queue out=w441:refnum<queue>, error out=w440:errorcluster)  [unwired: 1 in, 1 out]
      }
    }
    n226 = case shown="True" w206 {
      tunnel: w203 -> [w449 w454]
      tunnel: w202 -> [w448 w453]
      tunnel: [w449 w452] -> w199
      tunnel: [w448 w451] -> w198
      frame False {
      }
      frame True {
        # "Put \"Metal\" in the Queue"
        # "It is metal only"
        n227 = local read "Metal Count"() -> (w456:dbl)
        n228 = Increment(x=w456) -> (x+1=w455:dbl)
        n229 = local write "Metal Count"(w455) -> ()
        n230 = Enqueue Element(queue=w454, element="Metal", error in (no error)=w453) -> (queue out=w452:refnum<queue>, error out=w451:errorcluster)  [unwired: 1 in, 1 out]
      }
    }
    n231 = case shown="True" w181 {
      frame False {
      }
      frame True {
        n232 = flat-sequence {
          frame #0 {
            n233 = local read "Assembled"() -> (w337:dbl)
            n234 = local read "Plastic Count"() -> (w334:dbl)
            n235 = local read "Metal Count"() -> (w335:dbl)
            n236 = Multiply(x=w337, y=2.0) -> (x*y=w336:dbl)
            n237 = Add(x=w334, y=w335) -> (x+y=w333:dbl)
            n238 = Divide(x=w336, y=w333) -> (x/y=w332:dbl)
            n239 = Multiply(x=w332, y=100.0) -> (x*y=w330:dbl)
            n240 = local write "Efficiency"(w330) -> ()
          }
          frame #1 {
            n241 = local read "Efficiency"() -> (w339:dbl)
            n242 = local write "System Efficiency"(w339) -> ()
          }
        }
      }
    }
    n243 = call-poly <vilib>:"DAQmx Read.vi"("task/channels in"=w263, "error in"=w264) -> ("task out"=w260:refnum<k21>, "data"=→"Capacitive Sensor":bool, "error out"=w259:errorcluster)  [unwired: 11 in]
    n244 = call-poly <vilib>:"DAQmx Read.vi"("task/channels in"=w265, "error in"=w266) -> ("task out"=w258:refnum<k21>, "data"=→"Sensing - Metal Detector":bool, "error out"=w257:errorcluster)  [unwired: 11 in]
    n245 = call-poly <vilib>:"DAQmx Read.vi"("task/channels in"=w262, "error in"=w261) -> ("task out"=w252:refnum<k21>, "data"=→"Fibre Optic":bool, "error out"=w251:errorcluster)  [unwired: 11 in]
    n246 = call-poly <vilib>:"DAQmx Read.vi"("task/channels in"=w270, "error in"=w269) -> ("task out"=w254:refnum<k21>, "data"=→"Reject IR":bool, "error out"=w253:errorcluster)  [unwired: 11 in]
    n247 = case shown="True" w295 {
      frame False {
      }
      frame True {
        n248 = local write "Belt & Chain"(TRUE ("Boolean")) -> ()
      }
    }
    n249 = case shown="True" w179 {
      frame False {
      }
      frame True {
        n250 = local write "Stop"(FALSE) -> ()
        "Running" <- TRUE
      }
    }
    n251 = local read "# Elements in Queue"() -> (w185:i32)
    n252 = local read "Reject IR - Pos Edge"() -> (w186:bool)
    n253 = Greater Than 0?(x=w185) -> (x > 0?=w184:bool)
    n254 = And(x=w186, y=w184) -> (x .and. y?=w187:bool)
    n255 = case shown="True" w187 {
      tunnel: w199 -> [w412 w416]
      tunnel: w198 -> [w411 w415]
      tunnel: [w411 w414] -> w197
      tunnel: [w412 w413] -> w196
      frame False {
      }
      frame True {
        n256 = flat-sequence {
          tunnel: w416 -> [w421]
          tunnel: w415 -> [w420]
          tunnel: [w419] -> w414
          tunnel: [w418] -> w413
          frame #0 {
            # "Check Queue's first element"
            n257 = Dequeue Element(queue=w421, error in (no error)=w420) -> (queue out=w418:refnum<queue>, element=w417:string, error out=w419:errorcluster)  [unwired: 1 in, 1 out]
            n258 = local write "Dequeued Element"(w417) -> ()
          }
          frame #1 {
            n259 = local read "Dequeued Element"() -> (w425:string)
            n260 = local read "Dequeued Element"() -> (w429:string)
            n261 = local read "Dequeued Element"() -> (w430:string)
            n262 = Equal?(x=w429, y="Metal") -> (x = y?=w423:bool)
            n263 = Equal?(x=w425, y="Packaged") -> (x = y?=w424:bool)
            n264 = Equal?(x=w430, y="Plastic") -> (x = y?=w422:bool)
            n265 = case shown="True" w423 {
              frame False {
              }
              frame True {
                # "Kick Out"
                # "If Metal"
                n266 = local write "Reject Solenoid"(TRUE) -> ()
              }
            }
            n267 = case shown="True" w422 {
              frame False {
              }
              frame True {
                # "Kick Out"
                # "If Plastic"
                n268 = local write "Reject Solenoid"(TRUE) -> ()
              }
            }
            n269 = case shown="True" w424 {
              frame False {
              }
              frame True {
                # "Don't Kick out"
                # "If Packaged"
                n270 = local write "Reject Solenoid"(FALSE) -> ()
              }
            }
          }
        }
      }
    }
    n271 = local read "Plastic Count"() -> (→"Plastics":dbl)
    n272 = local read "Metal Count"() -> (→"Metals":dbl)
    n273 = local read "Assembled"() -> (→"Assembled":dbl)
    n274 = local read "Capacitive Sensor"() -> (w233:bool)
    n275 = local read "Rotary Solenoid"() -> (w237:bool)
    n276 = local read "Reject Solenoid"() -> (w192:bool)
    n277 = local read "Reject IR - Neg Edge"() -> (w193:bool)
    n278 = local read "Capacitive State"() -> (w217:bool)
    n279 = local read "Metal State 2"() -> (w221:bool)
    n280 = local read "Fibre Optic"() -> (w231:bool)
    n281 = local read "Reject IR"() -> (w200:bool)
    n282 = case shown="True" w193 {
      frame False {
      }
      frame True {
        n283 = local write "Reject Solenoid"(FALSE) -> ()
      }
    }
    n284 = call-poly <vilib>:"DAQmx Write.vi"("task/channels in"=w267, "data"=w192, "error in"=w268) -> ("task out"=w256:refnum<k21>, "error out"=w255:errorcluster)  [unwired: 10 in, 1 out]
    "Loop Iteration" <- w174
  }
  n285 = call <vilib>:"DAQmx Stop Task.vi"("task/channels in"=w42, "error in"=w41) -> ("task out"=w52:refnum<k21>, "error out"=w51:errorcluster)  [unwired: 12 in]
  n286 = call <vilib>:"DAQmx Stop Task.vi"("task/channels in"=w44, "error in"=w43) -> ("task out"=w50:refnum<k21>, "error out"=w49:errorcluster)  [unwired: 12 in]
  n287 = call <vilib>:"DAQmx Stop Task.vi"("task/channels in"=w38, "error in"=w37) -> ("task out"=w56:refnum<k21>, "error out"=w55:errorcluster)  [unwired: 12 in]
  n288 = call <vilib>:"DAQmx Stop Task.vi"("task/channels in"=w40, "error in"=w39) -> ("task out"=w54:refnum<k21>, "error out"=w53:errorcluster)  [unwired: 12 in]
  n289 = call <vilib>:"DAQmx Stop Task.vi"("task/channels in"=w46, "error in"=w45) -> ("task out"=w48:refnum<k21>, "error out"=w47:errorcluster)  [unwired: 12 in]
  n290 = call <vilib>:"DAQmx Stop Task.vi"("task/channels in"=w100, "error in"=w101) -> ("task out"=w155:refnum<k21>, "error out"=w154:errorcluster)  [unwired: 12 in]
  n291 = call <vilib>:"DAQmx Clear Task.vi"("task in"=w52, "error in"=w51) -> ()  [unwired: 13 in, 1 out]
  n292 = call <vilib>:"DAQmx Clear Task.vi"("task in"=w50, "error in"=w49) -> ()  [unwired: 13 in, 1 out]
  n293 = call <vilib>:"DAQmx Clear Task.vi"("task in"=w56, "error in"=w55) -> ()  [unwired: 13 in, 1 out]
  n294 = call <vilib>:"DAQmx Clear Task.vi"("task in"=w54, "error in"=w53) -> ()  [unwired: 13 in, 1 out]
  n295 = call <vilib>:"DAQmx Clear Task.vi"("task in"=w48, "error in"=w47) -> ()  [unwired: 13 in, 1 out]
  n296 = call <vilib>:"DAQmx Stop Task.vi"("task/channels in"=w142, "error in"=w143) -> ("task out"=w145:refnum<k21>, "error out"=w144:errorcluster)  [unwired: 12 in]
  n297 = call <vilib>:"DAQmx Stop Task.vi"("task/channels in"=w151, "error in"=w152) -> ("task out"=w159:refnum<k21>, "error out"=w158:errorcluster)  [unwired: 12 in]
  n298 = call <vilib>:"DAQmx Stop Task.vi"("task/channels in"=w4, "error in"=w3) -> ("task out"=w5:refnum<k21>, "error out"=w6:errorcluster)  [unwired: 12 in]
  n299 = call <vilib>:"DAQmx Stop Task.vi"("task/channels in"=w113, "error in"=w112) -> ("task out"=w115:refnum<k21>, "error out"=w114:errorcluster)  [unwired: 12 in]
  n300 = call <vilib>:"DAQmx Stop Task.vi"("task/channels in"=w29, "error in"=w28) -> ("task out"=w31:refnum<k21>, "error out"=w30:errorcluster)  [unwired: 12 in]
  n301 = call <vilib>:"DAQmx Stop Task.vi"("task/channels in"=w121, "error in"=w120) -> ("task out"=w123:refnum<k21>, "error out"=w122:errorcluster)  [unwired: 12 in]
  n302 = call <vilib>:"DAQmx Clear Task.vi"("task in"=w155, "error in"=w154) -> ()  [unwired: 13 in, 1 out]
  n303 = call <vilib>:"DAQmx Stop Task.vi"("task/channels in"=w130, "error in"=w129) -> ("task out"=w132:refnum<k21>, "error out"=w131:errorcluster)  [unwired: 12 in]
  n304 = Flush Queue(queue=w20, error in (no error)=w17) -> (queue out=w19:refnum<queue>, error out=w18:errorcluster)  [unwired: 1 out]
  n305 = call <vilib>:"DAQmx Clear Task.vi"("task in"=w145, "error in"=w144) -> ()  [unwired: 13 in, 1 out]
  n306 = call <vilib>:"DAQmx Clear Task.vi"("task in"=w159, "error in"=w158) -> ()  [unwired: 13 in, 1 out]
  n307 = Release Queue(queue=w19, error in (no error)=w18) -> ()  [unwired: 1 in, 3 out]
  n308 = call <vilib>:"DAQmx Stop Task.vi"("task/channels in"=w102, "error in"=w103) -> ("task out"=w110:refnum<k21>, "error out"=w109:errorcluster)  [unwired: 12 in]
  n309 = call <vilib>:"DAQmx Stop Task.vi"("task/channels in"=w92, "error in"=w91) -> ("task out"=w94:refnum<k21>, "error out"=w93:errorcluster)  [unwired: 12 in]
  n310 = call <vilib>:"DAQmx Stop Task.vi"("task/channels in"=w82, "error in"=w83) -> ("task out"=w90:refnum<k21>, "error out"=w89:errorcluster)  [unwired: 12 in]
  n311 = call <vilib>:"DAQmx Clear Task.vi"("task in"=w5, "error in"=w6) -> ()  [unwired: 13 in, 1 out]
  n312 = call <vilib>:"DAQmx Clear Task.vi"("task in"=w115, "error in"=w114) -> ()  [unwired: 13 in, 1 out]
  n313 = call <vilib>:"DAQmx Clear Task.vi"("task in"=w31, "error in"=w30) -> ()  [unwired: 13 in, 1 out]
  n314 = call <vilib>:"DAQmx Clear Task.vi"("task in"=w123, "error in"=w122) -> ()  [unwired: 13 in, 1 out]
  n315 = call <vilib>:"DAQmx Clear Task.vi"("task in"=w132, "error in"=w131) -> ()  [unwired: 13 in, 1 out]
  n316 = call <vilib>:"DAQmx Clear Task.vi"("task in"=w110, "error in"=w109) -> ()  [unwired: 13 in, 1 out]
  n317 = call <vilib>:"DAQmx Clear Task.vi"("task in"=w94, "error in"=w93) -> ()  [unwired: 13 in, 1 out]
  n318 = call <vilib>:"DAQmx Clear Task.vi"("task in"=w90, "error in"=w89) -> ()  [unwired: 13 in, 1 out]
  "Capacitive State" <- w25
  "Sort Solenoid" <- w26
  "Rotary Solenoid" <- FALSE
  "Metal State" <- w26
  "Metal State 2" <- w25
  "Sensing - Plastic State" <- w25
  "Metal Count" <- w15
  "Plastic Count" <- w12
  "Reject Solenoid" <- w25
  "Belt & Chain" <- FALSE ("Conveyor Belt")
  "# Elements in Queue" <- w15
  "File Read" <- FALSE
  "Hopper \nCount" <- 0 ("# of Plastics in \nAssembly Chute")
  "Assembled" <- w12
  "Efficiency" <- w10
  "Dequeued Element" <- " " ("Dequeued Element")
  "System Efficiency" <- w10
